vi "set memory.vi"(8 "error in (no error)":errorcluster caption="에러 입력(에러 없음)", 10 "WF List":T1[](array[typedef]), 11 "DW7914 입력":refnum<class "DW7914.lvclass">) -> (0 "error out":errorcluster caption="에러 출력", 3 "DW7914 출력":refnum<class "DW7914.lvclass">)   [LabVIEW 2020, in "DW7914.lvclass"]
uses:
  DW7914.lvclass
  SubVIs/Waveform Editor/Controls/(Ctrl)Waveform Editor_WF List.ctl
  Waveform Obj Class/Waveform Obj/Waveform Obj.lvclass
  Haptic IC/Haptic IC.lvclass/Haptic IC.ctl
  SubVIs/I2C/Instance VIs/(SubVI)I2C_8Bit-8Bit_Read_Single.vi
  SubVIs/I2C/Instance VIs/(SubVI)I2C_8Bit-8Bit_Write_Single.vi
  SubVIs/I2C/Instance VIs/(SubVI)I2C_8Bit-8Bit_Write_Sequential.vi
  DW7914.lvclass/DW7914.ctl
  Haptic IC/Haptic IC.lvclass
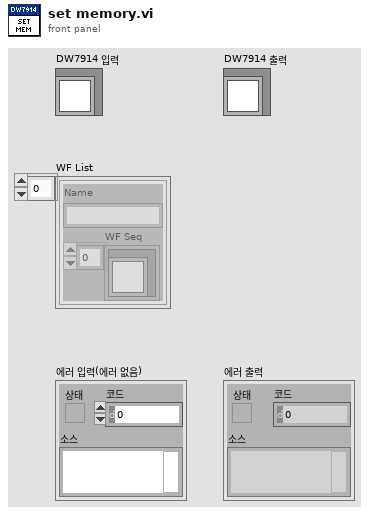
[diagram p1: front panel]
types:
  T1 = typedef "(Ctrl)Waveform Editor_WF List.ctl" = cluster{"Name":string, "WF Seq":refnum<class "Waveform Obj.lvclass">[]}
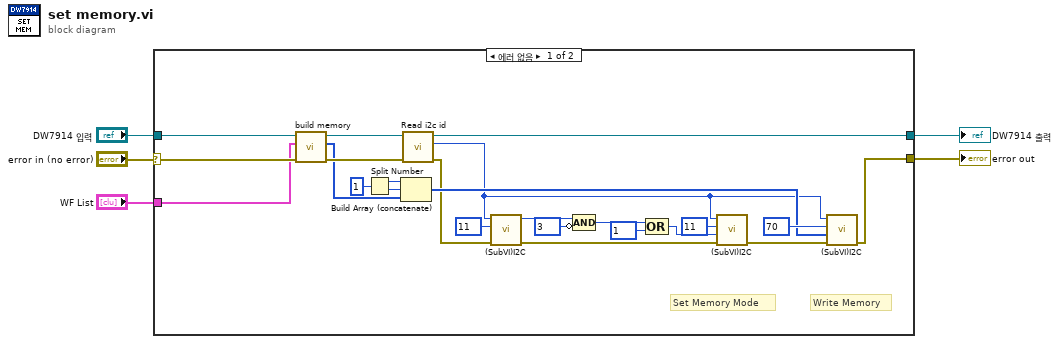
[diagram p0: block diagram]
diagram:
  n1 = case shown="에러 없음" "error in (no error)" {
    selector: "error in (no error)" -> [w22 w31]
    tunnel: [w23 w31] -> w5
    tunnel: "DW7914 입력" -> [w20 w30]
    tunnel: [w29 w30] -> w4
    tunnel: "WF List" -> [w18 _]
    frame No Error {
      # "Write Memory"
      # "Set Memory Mode"
      n2 = call-dynamic "build memory.vi"("error in (no error)"=w22, "WF List"=w18, "DW7912 입력"=w20) -> ("error out"=w21:errorcluster, "full memory data"=w17:u8[], "DW7912 출력"=w19:refnum<class "DW7914.lvclass">)  [unwired: 5 in, 1 out]
      n3 = Split Number(x=u16 1) -> (hi(x)=w26:u8, lo(x)=w25:u8)
      n4 = Build Array (concatenate)(w26, w25, w17) -> (w24:u8[])
      n5 = call "Read i2c id.vi"("error in (no error)"=w21, "Haptic IC 입력"=w19) -> ("error out"=w9:errorcluster, "i2c id"=w8:u8, "Haptic IC 출력"=w29:refnum<class "DW7914.lvclass">)  [unwired: 7 in]
      n6 = call-poly "(SubVI)I2C.vi"("error in (no error)"=w9, "Address"=u8 11, "ID"=w8) -> ("error out"=w15:errorcluster, "Read Data"=w16:u8)  [unwired: 6 in, 1 out]
      n7 = Compound Arithmetic op=AND(w16, invert u8 3 ("y")) -> (w7:u8)
      n8 = Compound Arithmetic op=OR(w7, u8 1 ("y")) -> (w14:u8)
      n9 = call-poly "(SubVI)I2C.vi"("error in (no error)"=w15, "Data to Write"=w14, "Address"=u8 11, "ID"=w8) -> ("error out"=w10:errorcluster)  [unwired: 6 in, 1 out]
      n10 = call-poly "(SubVI)I2C.vi"("error in (no error)"=w10, "Data to Write"=w24, "Start Address"=u8 70, "ID"=w8) -> ("error out"=w23:errorcluster)  [unwired: 6 in, 1 out]
    }
    frame Error {
    }
  }
  "error out" <- w5
  "DW7914 출력" <- w4
